vi "TestRUSHShoot.vi"() -> ()   [LabVIEW 2012]
panel:
  in  "ShootRollerSpd":dbl(slide) scale=-1.0..1.0
  in  "In Cluster":T1
  in  "Ground":bool
  in  "Set 4":bool
  in  "ShootConstElev":T2={"1"=2.0, "2"=3.0, "3"=3.5, "4"=4.0, "Ground"=1.0}
  out "Out Cluster":T3
  in  "Set 3":bool
  in  "Set 2":bool
  in  "Set 1":bool
  in  "ShootTargetInfo":T4
  in  "Deadband":dbl=0.1
  in  "Default Wheel Speed":dbl=0.75
  in  "IndexerSpeed":dbl=0.5
  in  "ShootManualElev":dbl(slide) scale=-1.0..1.0
  in  "ShootPOTElev":dbl(slide) scale=0.0..5.0
  in  "ShootIndexerEnable":bool
  in  "ShootStartWheels":bool
  in  "ShootTrackEnable":bool
  # "Roller Speed IN"
  # "Roller OUT"
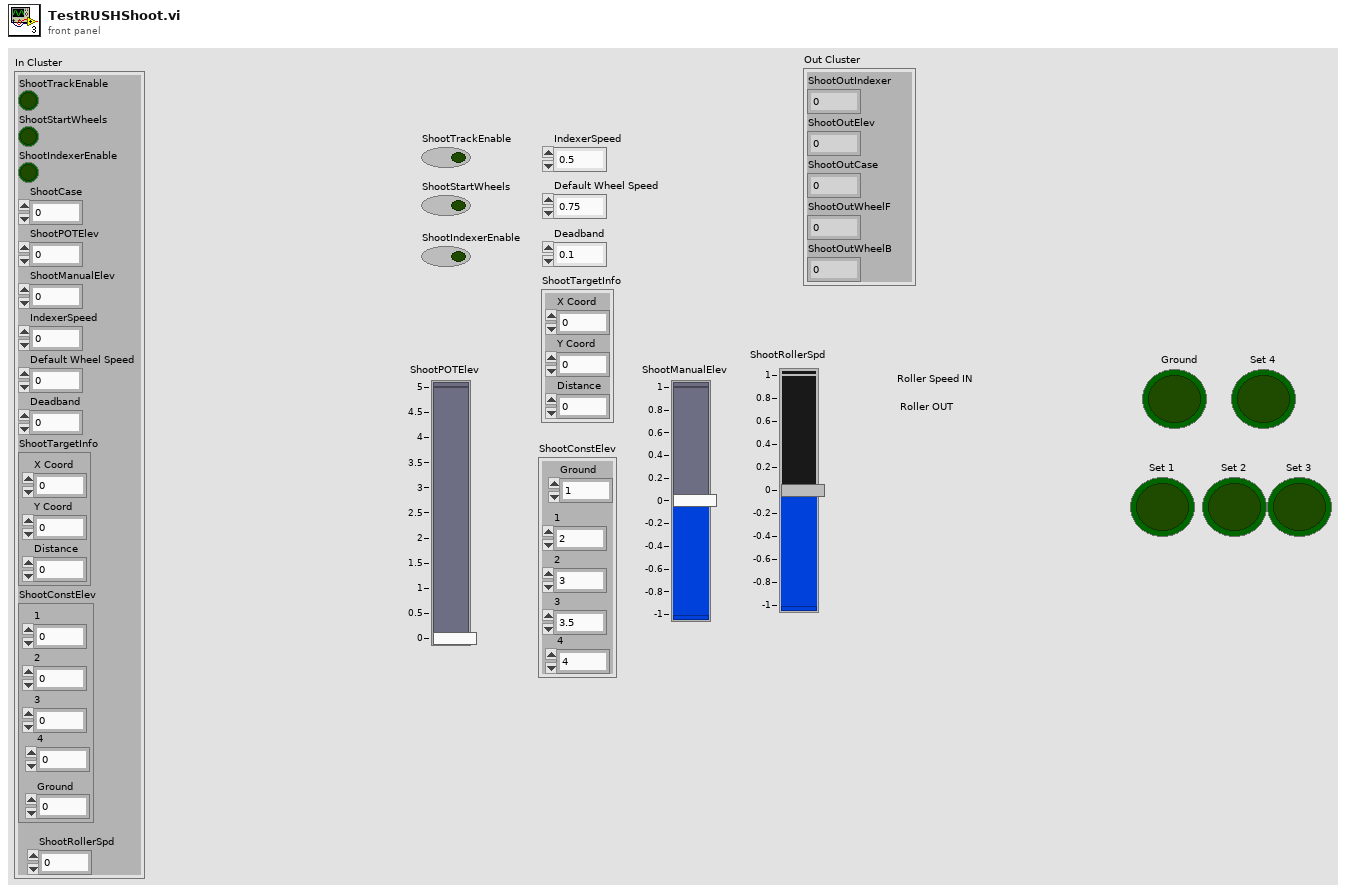
[diagram p1: front panel]
types:
  T1 = cluster{"ShootTrackEnable":bool, "ShootStartWheels":bool, "ShootIndexerEnable":bool, "ShootCase":dbl, "ShootPOTElev":dbl, "ShootManualElev":dbl, "IndexerSpeed":dbl, "Default Wheel Speed":dbl, "Deadband":dbl, "ShootTargetInfo":cluster{"X Coord":dbl, "Y Coord":dbl, "Distance":dbl}, "ShootConstElev":cluster{"1":dbl, "2":dbl, "3":dbl, "4":dbl, "Ground":dbl}, "ShootRollerSpd":dbl}
  T2 = cluster{"1":dbl, "2":dbl, "3":dbl, "4":dbl, "Ground":dbl}
  T3 = cluster{"ShootOutIndexer":dbl, "ShootOutElev":dbl, "ShootOutCase":dbl, "ShootOutWheelF":dbl, "ShootOutWheelB":dbl}
  T4 = cluster{"X Coord":dbl, "Y Coord":dbl, "Distance":dbl}
  T5 = cluster{"ShootOutIndexer":dbl, "ShootOutElev":dbl, "ShootOutCase":dbl, "ShootOutWheelF":dbl, "ShootOutRollers":dbl}
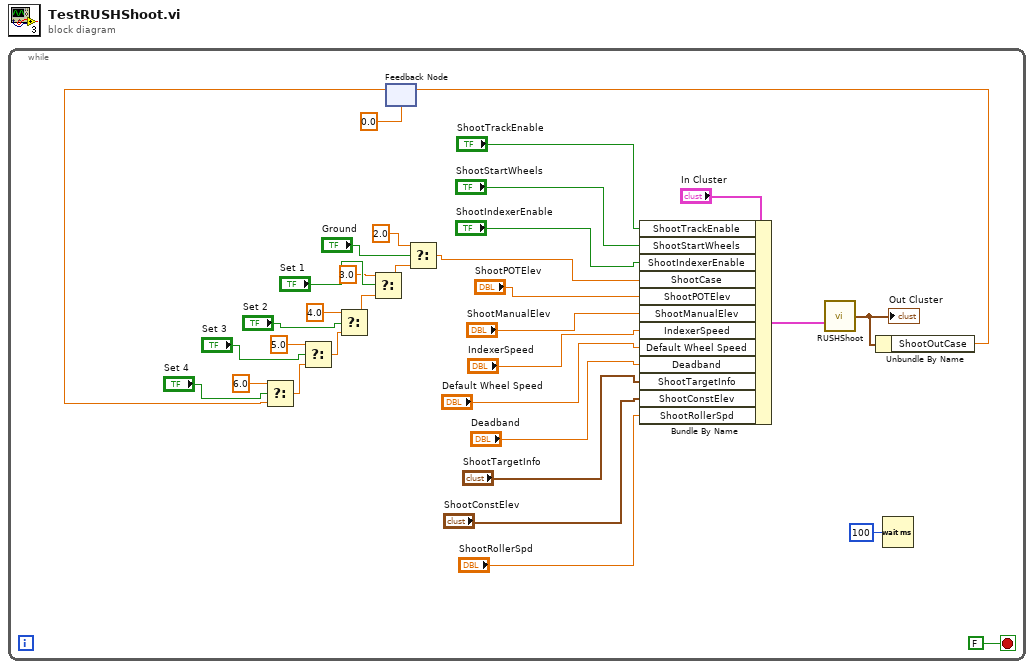
[diagram p0: block diagram]
diagram:
  n1 = while {
    stop <- FALSE stop-if-true
    n2 = feedback #1(0.0 ("ShootOutCase")) -> (w5:dbl)
    n3 = Select(t=6.0, s="Set 4", f=w5) -> (s? t:f=w11:dbl)
    n4 = Select(t=5.0, s="Set 3", f=w11) -> (s? t:f=w30:dbl)
    n5 = Select(t=4.0, s="Set 2", f=w30) -> (s? t:f=w29:dbl)
    n6 = Select(t=3.0, s="Set 1", f=w29) -> (s? t:f=w7:dbl)
    n7 = Select(t=2.0, s="Ground", f=w7) -> (s? t:f=w10:dbl)
    n8 = Bundle By Name(cluster="In Cluster", "ShootTrackEnable"="ShootTrackEnable", "ShootStartWheels"="ShootStartWheels", "ShootIndexerEnable"="ShootIndexerEnable", "ShootCase"=w10, "ShootPOTElev"="ShootPOTElev", "ShootManualElev"="ShootManualElev", "IndexerSpeed"="IndexerSpeed", "Default Wheel Speed"="Default Wheel Speed", "Deadband"="Deadband", "ShootTargetInfo"="ShootTargetInfo", "ShootConstElev"="ShootConstElev", "ShootRollerSpd"="ShootRollerSpd") -> (w2:T1)
    n9 = call "RUSHShoot.vi"("In Cluster"=w2) -> ("Out Cluster"=w16:T5)
    "Out Cluster" <- w16
    n10 = Unbundle By Name(w16) -> ("ShootOutCase"=w6:dbl)
    n11 = feedback-in #1(w6) -> ()
    n12 = Wait (ms)(milliseconds to wait=u32 100) -> ()  [unwired: 1 out]
  }
